vi "FIlter Selection.vi"(11 "Measuring Wavelength":dbl format="%#.7f nm") -> (3 "Filter Num":i32=1 min=1 max=5 step=1)   [LabVIEW 2021]
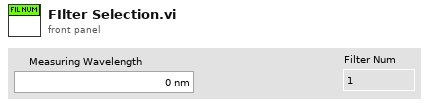
[diagram p1: front panel]
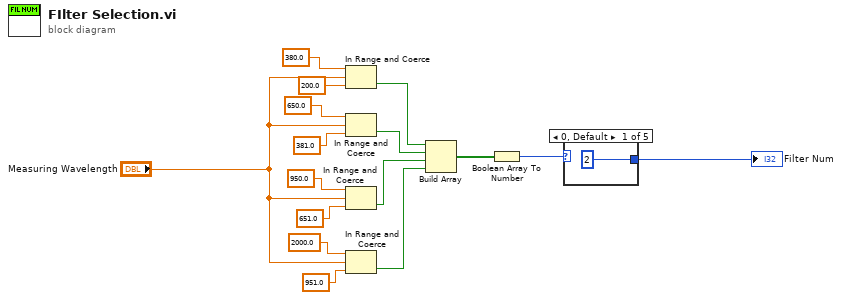
[diagram p0: block diagram]
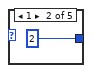
[diagram p2: hidden frame]
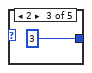
[diagram p3: hidden frame]
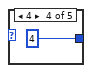
[diagram p4: hidden frame]
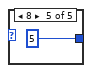
[diagram p5: hidden frame]
diagram:
  n1 = In Range and Coerce(upper limit=380.0, x="Measuring Wavelength", lower limit=200.0) -> (In Range?=w8:bool)  [unwired: 1 out]
  n2 = In Range and Coerce(upper limit=650.0, x="Measuring Wavelength", lower limit=381.0) -> (In Range?=w7:bool)  [unwired: 1 out]
  n3 = In Range and Coerce(upper limit=950.0, x="Measuring Wavelength", lower limit=651.0) -> (In Range?=w6:bool)  [unwired: 1 out]
  n4 = In Range and Coerce(upper limit=2000.0, x="Measuring Wavelength", lower limit=951.0) -> (In Range?=w5:bool)  [unwired: 1 out]
  n5 = Build Array(w8, w7, w6, w5) -> (w4:bool[])
  n6 = Boolean Array To Number(Boolean array=w4) -> (number=w3:u32)
  n7 = case shown="0, Default" w3 {
    tunnel: [2 ("Filter Num") 2 ("Filter Num") 3 ("Filter Num") 4 ("Filter Num") 5 ("Filter Num")] -> w1
    frame 0, Default {
    }
    frame 1 {
    }
    frame 2 {
    }
    frame 4 {
    }
    frame 8 {
    }
  }
  "Filter Num" <- w1
